vi "peelFileCheck.vi"() -> ()   [LabVIEW 2012]
uses:
  <vilib>/addons/database/Connection.llb/DB Tools Open Connec (Path).vi
  <vilib>/addons/database/Connection.llb/Conn Execute.vi
  <vilib>/addons/database/Recordset.llb/Rec Fetch Recordset Data (R).vi
  <vilib>/addons/database/Recordset.llb/Rec Destroy - Connection.vi
  <vilib>/addons/database/_DB Variant To Data/Database Variant To Data.xnode
  <vilib>/addons/database/NI_Database_API.lvlib
  <vilib>/Utility/SMTP/NI_SMTPEmail.lvlib
panel:
  out "spreadsheet string":string
  out "array":string[][](array[string])
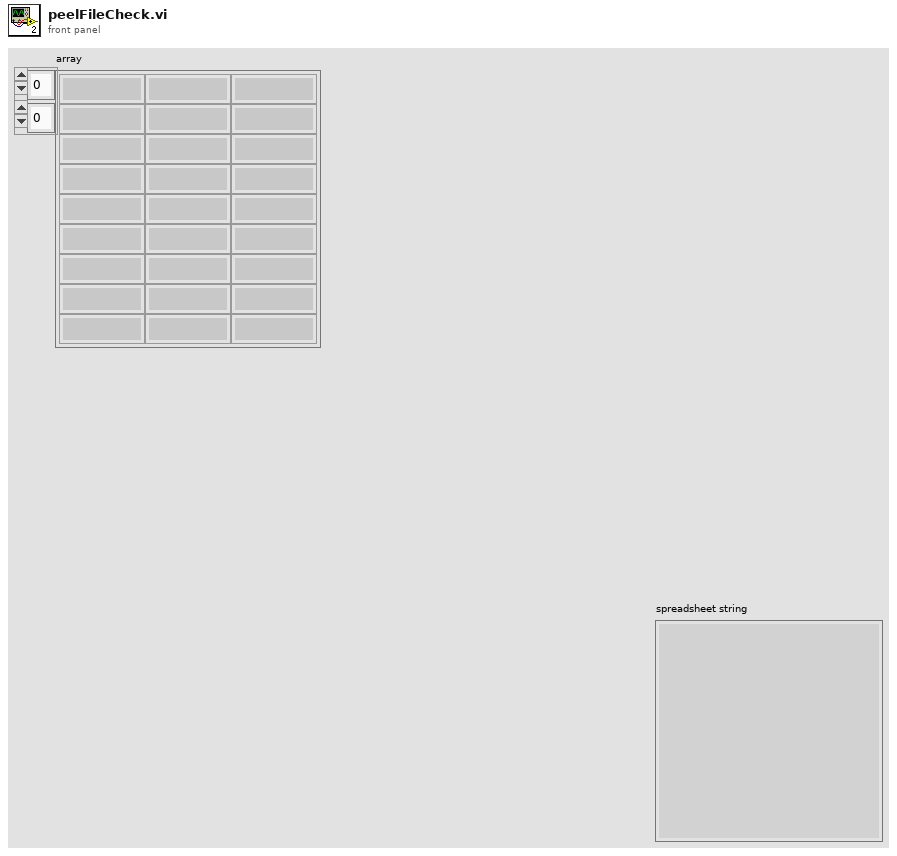
[diagram p1: front panel]
types:
  T1 = typedef "NI_Database_API.lvlib/Conn ObjectReference.ctl" = refnum<k1>
  T2 = typedef "NI_Database_API.lvlib/Rec ObjectReference.ctl" = refnum<k1>
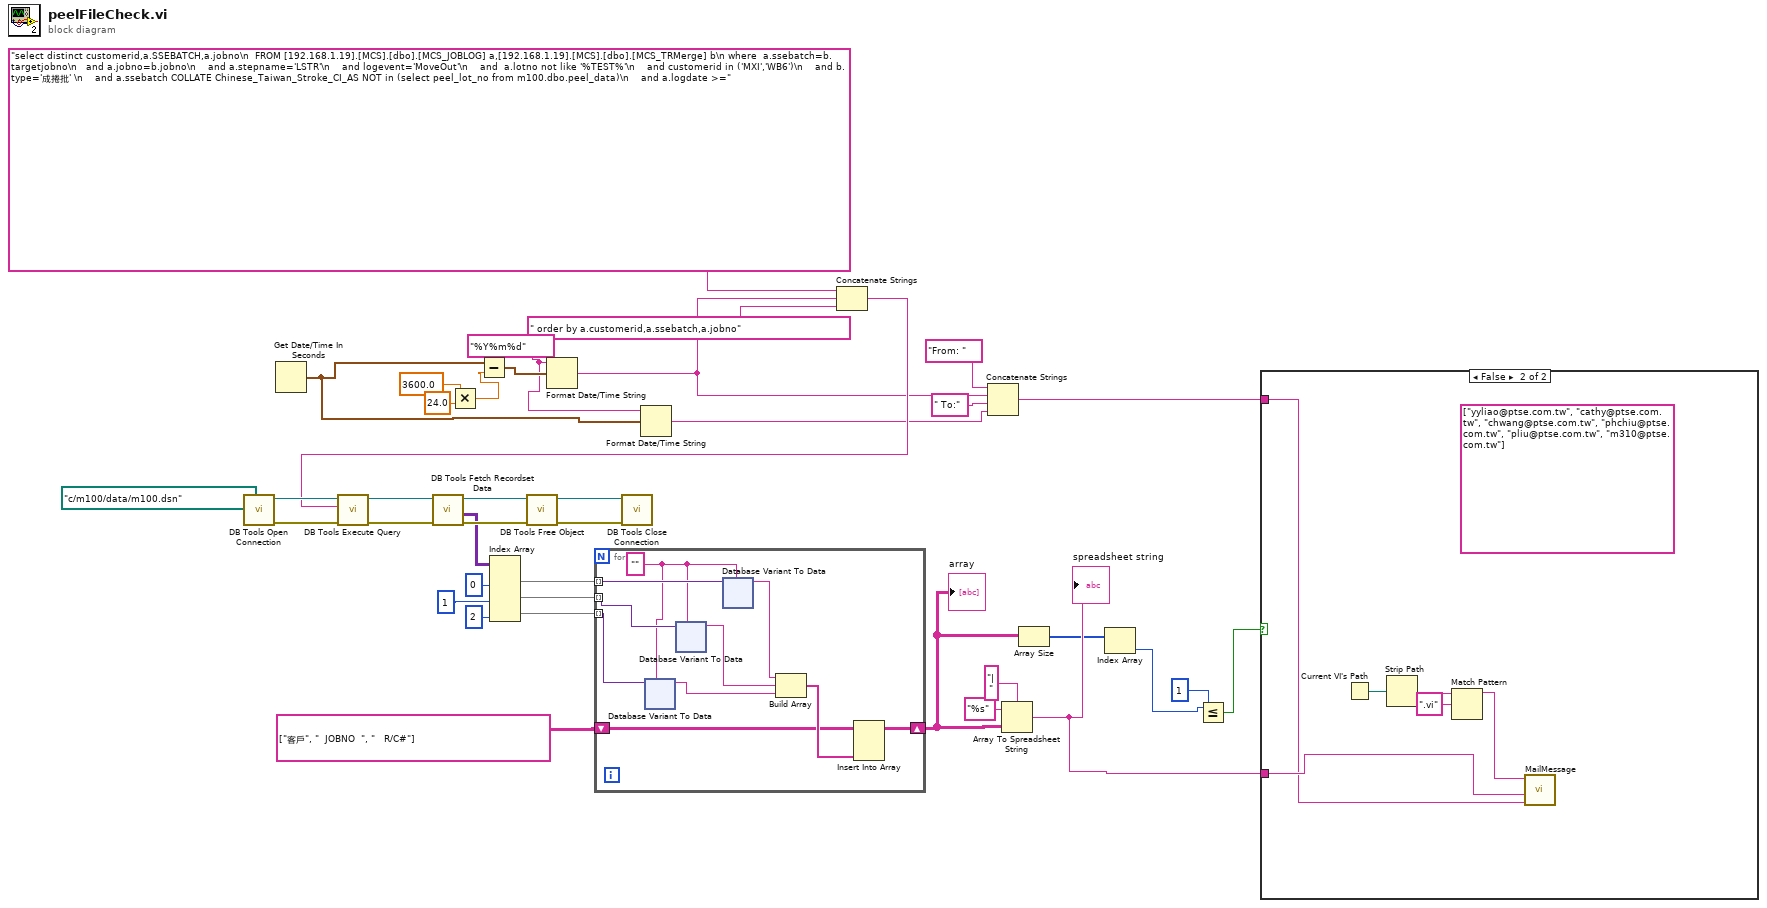
[diagram p0: block diagram]
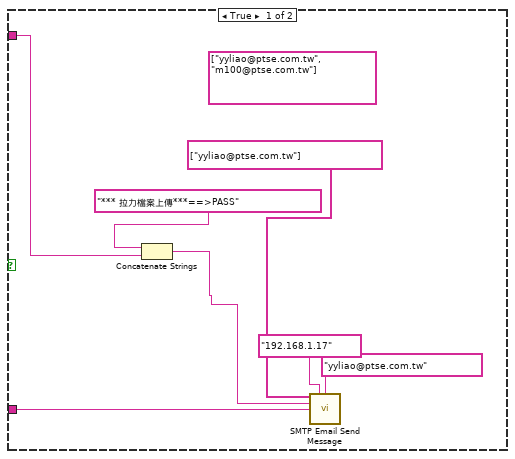
[diagram p2: hidden frame]
diagram:
  w9 = "%Y%m%d" ("time format string (%c)")
  n1 = call-poly <vilib>:"DB Tools Open Connection.vi"("connection information"=path "c:/m100/data/m100.dsn") -> ("error out"=w35:errorcluster, "connection reference"=w39:T1)  [unwired: 7 in]
  n2 = Get Date/Time In Seconds() -> (seconds since 1Jan1904=w10:timestamp)
  n3 = Multiply(x=3600.0, y=24.0) -> (x*y=w15:dbl)
  n4 = Subtract(x=w10, y=w15) -> (x-y=w13:timestamp)
  n5 = Format Date/Time String(time format string (%c)=w9, seconds (now)=w13) -> (date/time string=w7:string)  [unwired: 1 in]
  n6 = Format Date/Time String(time format string (%c)=w9, seconds (now)=w10) -> (date/time string=w5:string)  [unwired: 1 in]
  n7 = Concatenate Strings("select distinct customerid,a.SSEBATCH,a.jobno\n  FROM [192.168.1.19].[MCS].[dbo].[MCS_JOBLOG] a,[192.168.1.19].[MCS].[dbo].[MCS_TRMerge] b\n where  a.ssebatch=b.targetjobno\n   and a.jobno=b.jobno\n    and a.stepname='LSTR'\n    and logevent='MoveOut'\n    and  a.lotno not like '%TEST%'\n    and customerid in ('MXI','WB6')\n    and b.type='成捲批' \n    and a.ssebatch COLLATE Chinese_Taiwan_Stroke_CI_AS NOT in (select peel_lot_no from m100.dbo.peel_data)\n    and a.logdate >=", w7, " order by a.customerid,a.ssebatch,a.jobno" ("string")) -> (w11:string)
  n8 = call-poly <vilib>:"DB Tools Execute Query.vi"("error in (no error)"=w35, "SQL query"=w11, "connection reference"=w39) -> ("error out"=w34:errorcluster, "recordset reference"=w38:T2)  [unwired: 5 in]
  n9 = call-poly <vilib>:"DB Tools Fetch Recordset Data.vi"("error in (no error)"=w34, "recordset reference"=w38) -> ("error out"=w33:errorcluster, "recordset data"=w30:variant[][], "recordset reference out"=w37:T2)  [unwired: 3 in]
  n10 = Index Array(array=w30, index (col) #1=0 ("disabled index (col)"), index (col) #2=1 ("disabled index (row)"), index (col) #3=2 ("disabled index (col)")) -> (element #1=w26:variant[], element #2=w25:variant[], element #3=w24:variant[])  [unwired: 3 in]
  n11 = call-poly <vilib>:"DB Tools Free Object.vi"("error in (no error)"=w33, "recordset reference"=w37) -> ("error out"=w32:errorcluster, "connection reference"=w36:T1)  [unwired: 8 in]
  n12 = for {
    tunnel: w26 -> [w49] mode=indexing
    tunnel: w25 -> [w48] mode=indexing
    tunnel: w24 -> [w47] mode=indexing
    shift-right: [w41] -> w3
    shift-left: string[][] [["客戶", "  JOBNO  ", "   R/C#"]] ("array") -> [w40]
    w46 = ""
    n13 = xnode "Database Variant To Data"("database variant"=w47, "type"=w46) -> ("data"=w43:string)  [unwired: 1 in, 1 out]
    n14 = xnode "Database Variant To Data"("database variant"=w48, "type"=w46) -> ("data"=w44:string)  [unwired: 1 in, 1 out]
    n15 = xnode "Database Variant To Data"("database variant"=w49, "type"=w46) -> ("data"=w45:string)  [unwired: 1 in, 1 out]
    n16 = Build Array(w45, w44, w43) -> (w42:string[])
    n17 = Insert Into Array(array=w40, new element=w42) -> (w41:string[][])  [unwired: 2 in]
  }
  "array" <- w3
  n18 = call <vilib>:"DB Tools Close Connection.vi"("error in (no error)"=w32, "connection reference"=w36) -> ()  [unwired: 5 in, 1 out]
  n19 = Concatenate Strings("From: " ("string"), w7, " To:" ("string"), w5) -> (w4:string)
  n20 = Array To Spreadsheet String(delimiter (Tab)="| ", array=w3, 3:"%s" ("format string")) -> (spreadsheet string=w18:string)
  "spreadsheet string" <- w18
  n21 = Array Size(array=w3) -> (size(s)=w2:i32[])
  n22 = Index Array(array=w2) -> (element=w1:i32)  [unwired: 1 in]
  n23 = Less Or Equal?(x=w1, y=1) -> (x <= y?=w19:bool)
  n24 = case shown="False" w19 {
    tunnel: w18 -> [w150 w154]
    tunnel: w4 -> [w146 w153]
    frame True {
      (unwired) string[] ["yyliao@ptse.com.tw", "m100@ptse.com.tw"] ("recipients")
      n25 = Concatenate Strings("*** 拉力檔案上傳***==>PASS" ("subject ([No Subject])"), w146) -> (w147:string)
      n26 = call <vilib>:"SMTP Email Send Message.vi"("recipients"=string[] ["yyliao@ptse.com.tw"], "mail server"="192.168.1.17", "return address"="yyliao@ptse.com.tw", "subject ([No Subject])"=w147, "message"=w150) -> ()  [unwired: 9 in, 2 out]
    }
    frame False {
      (unwired) string[] ["yyliao@ptse.com.tw", "cathy@ptse.com.tw", "chwang@ptse.com.tw", "phchiu@ptse.com.tw", "pliu@ptse.com.tw", "m310@ptse.com.tw"] ("recipients")
      n27 = Current VI's Path() -> (path=w158:path)
      n28 = Strip Path(path=w158) -> (name=w157:string)  [unwired: 1 out]
      n29 = Match Pattern(string=w157, regular expression=".vi") -> (before substring=w155:string)  [unwired: 1 in, 3 out]
      n30 = call "MailMessage.vi"("AddSubject"=w153, "message"=w154, "program"=w155) -> ()  [unwired: 9 in]
    }
  }
